vi "Log Data Core.vi"(8 "Error In":errorcluster, 10 "Log Message":T1={"Log Action"=enum."Handle Old Files", "Variant"=variant, "Data Type"=enum."String", "Group Name"="", "Channels Names"=[]}, 11 "TDMS Log In":refnum<class "TDMS Logger.lvclass">) -> (0 "Error Out":errorcluster, 3 "TDMS Log Out":refnum<class "TDMS Logger.lvclass">)   [LabVIEW 2015, in "TDMS Logger.lvlib" / "TDMS Logger.lvclass"]
uses:
  TDMS Logger.lvclass
  _Typedefs/Log Message.ctl
  _Typedefs/Log Action.ctl
  _Typedefs/Data Type.ctl
  TDMS Logger.lvclass/TDMS Logger.ctl
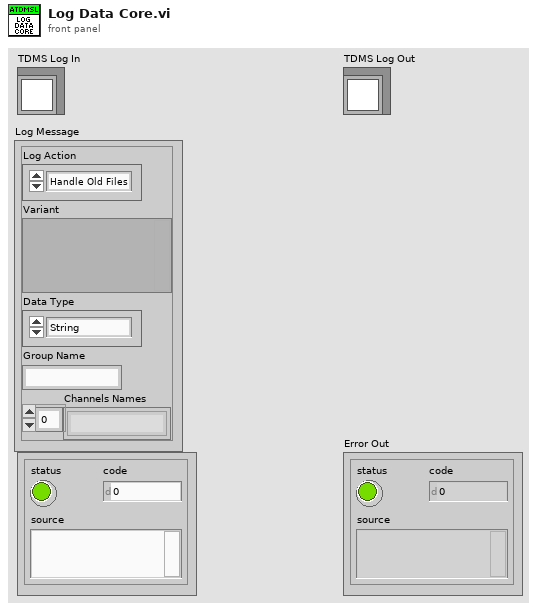
[diagram p1: front panel]
types:
  T1 = typedef "TDMS Logger.lvlib/TDMS Logger.lvclass/Log Message.ctl" = cluster{"Log Action":T2, "Variant":variant, "Data Type":T3, "Group Name":string, "Channels Names":string[]}
  T2 = typedef "TDMS Logger.lvlib/TDMS Logger.lvclass/Log Action.ctl" = enum16{"Handle Old Files", "Status Update", "Stop", "Log Data", "Initialize"}
  T3 = typedef "TDMS Logger.lvlib/TDMS Logger.lvclass/Data Type.ctl" = enum16{"I16", "I8", "String", "U16", "U8", "Waveform", "Double", "Single"}
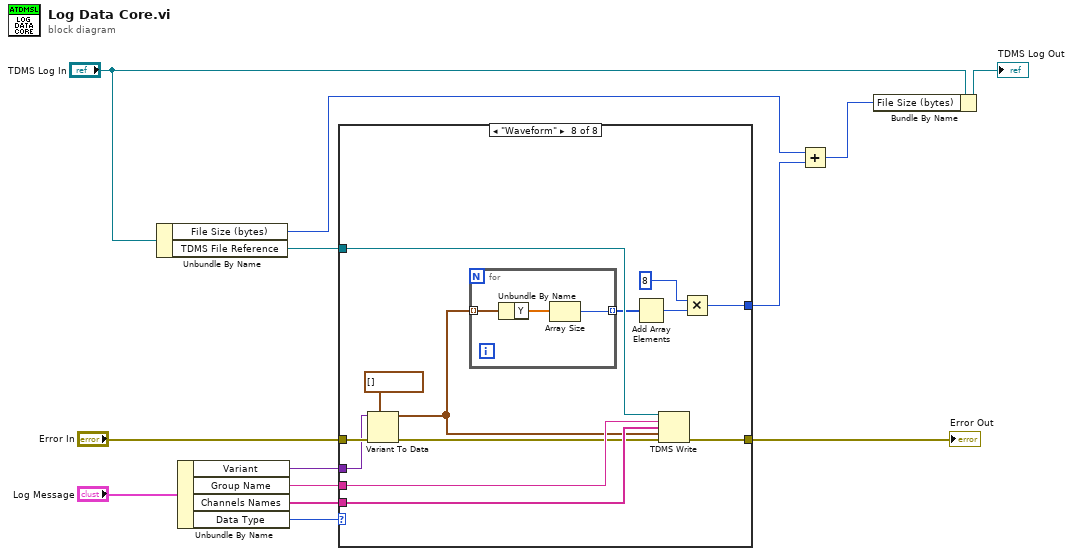
[diagram p0: block diagram]
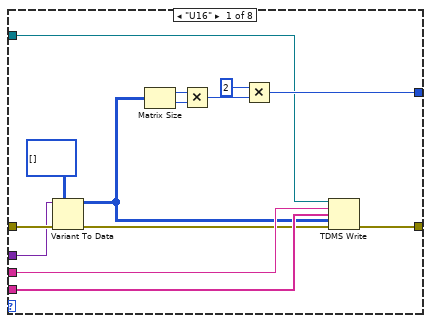
[diagram p2: hidden frame]
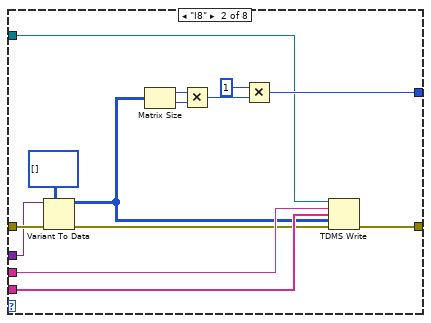
[diagram p3: hidden frame]
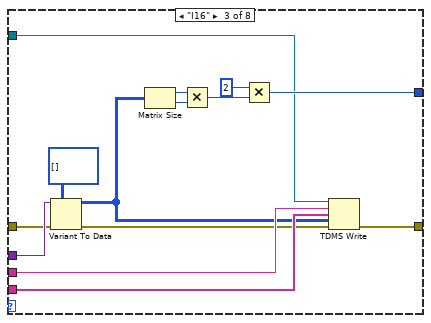
[diagram p4: hidden frame]
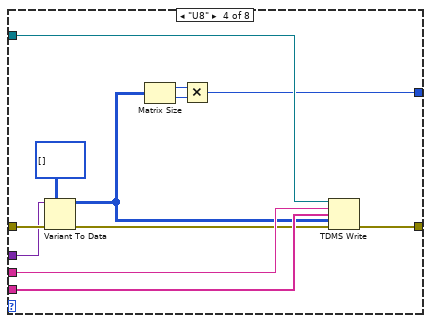
[diagram p5: hidden frame]
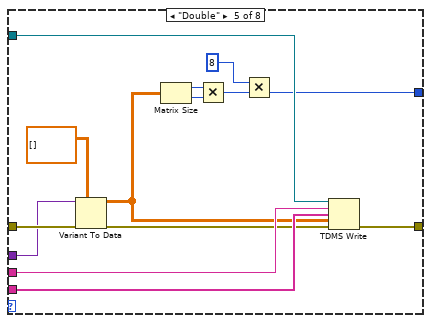
[diagram p6: hidden frame]
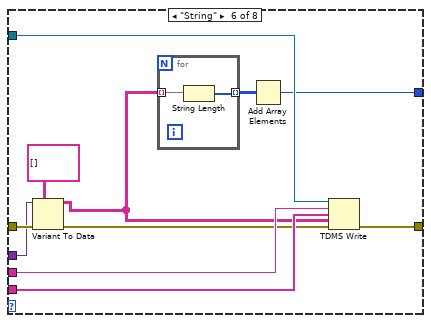
[diagram p7: hidden frame]
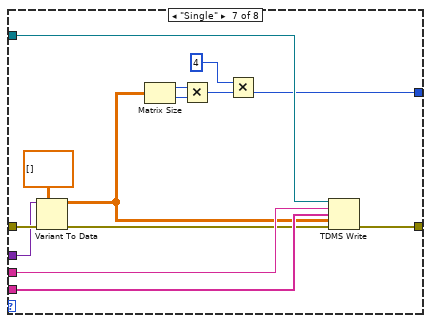
[diagram p8: hidden frame]
diagram:
  n1 = Unbundle By Name("TDMS Log In") -> ("File Size (bytes)"=w2:u64, "TDMS File Reference"=w4:refnum<k34>)
  n2 = Unbundle By Name("Log Message") -> ("Variant"=w1:variant, "Group Name"=w6:string, "Channels Names"=w5:string[], "Data Type"=w9:T3)
  n3 = case shown="\"Waveform\"" w9 {
    tunnel: "Error In" -> [w18 w32 w43 w60 w72 w86 w99 w113]
    tunnel: [w23 w41 w55 w61 w74 w87 w101 w117] -> w7
    tunnel: w6 -> [w22 w40 w54 w65 w79 w92 w106 w121]
    tunnel: w5 -> [w21 w39 w53 w64 w78 w91 w105 w120]
    tunnel: w4 -> [w20 w38 w52 w63 w77 w90 w104 w119]
    tunnel: [w19 w37 w51 w62 w76 w89 w103 w118] -> w3
    tunnel: w1 -> [w16 w28 w44 w56 w71 w82 w98 w109]
    frame "U16" {
      n4 = Variant To Data(error in=w18, type=u16[][] [] ("element"), Variant=w16) -> (data=w14:u16[][], error out=w17:errorcluster)
      n5 = Matrix Size(0:w14) -> (1:w25:i32, 2:w26:i32)
      n6 = Multiply(x=w25, y=w26) -> (x*y=w24:i32)
      n7 = Multiply(x=2, y=w24) -> (x*y=w23:i32)
      n8 = TDMS Write(0:w20, 5:w22, 7:w21, 9:w14, 11:w17) -> (15:w19:errorcluster)  [unwired: 1 in, 3 out]
    }
    frame "I8" {
      n9 = Variant To Data(error in=w32, type=i8[][] [] ("element"), Variant=w28) -> (data=w29:i8[][], error out=w31:errorcluster)
      n10 = Matrix Size(0:w29) -> (1:w34:i32, 2:w35:i32)
      n11 = Multiply(x=w34, y=w35) -> (x*y=w33:i32)
      n12 = Multiply(x=1, y=w33) -> (x*y=w41:i32)
      n13 = TDMS Write(0:w38, 5:w40, 7:w39, 9:w29, 11:w31) -> (15:w37:errorcluster)  [unwired: 1 in, 3 out]
    }
    frame "I16" {
      n14 = Variant To Data(error in=w43, type=i16[][] [] ("element"), Variant=w44) -> (data=w46:i16[][], error out=w42:errorcluster)
      n15 = Matrix Size(0:w46) -> (1:w48:i32, 2:w49:i32)
      n16 = Multiply(x=w48, y=w49) -> (x*y=w47:i32)
      n17 = Multiply(x=2, y=w47) -> (x*y=w55:i32)
      n18 = TDMS Write(0:w52, 5:w54, 7:w53, 9:w46, 11:w42) -> (15:w51:errorcluster)  [unwired: 1 in, 3 out]
    }
    frame "U8" {
      n19 = Variant To Data(error in=w60, type=u8[][] [] ("element"), Variant=w56) -> (data=w57:u8[][], error out=w59:errorcluster)
      n20 = Matrix Size(0:w57) -> (1:w66:i32, 2:w67:i32)
      n21 = Multiply(x=w66, y=w67) -> (x*y=w61:i32)
      n22 = TDMS Write(0:w63, 5:w65, 7:w64, 9:w57, 11:w59) -> (15:w62:errorcluster)  [unwired: 1 in, 3 out]
    }
    frame "Double" {
      n23 = Variant To Data(error in=w72, type=dbl[][] [], Variant=w71) -> (data=w68:dbl[][], error out=w70:errorcluster)
      n24 = Matrix Size(0:w68) -> (1:w80:i32, 2:w81:i32)
      n25 = Multiply(x=w80, y=w81) -> (x*y=w75:i32)
      n26 = Multiply(x=8, y=w75) -> (x*y=w74:i32)
      n27 = TDMS Write(0:w77, 5:w79, 7:w78, 9:w68, 11:w70) -> (15:w76:errorcluster)  [unwired: 1 in, 3 out]
    }
    frame "String" {
      n28 = Variant To Data(error in=w86, type=string[][] [] ("element"), Variant=w82) -> (data=w83:string[][], error out=w85:errorcluster)
      n29 = for {
        tunnel: w83 -> [w94] mode=indexing
        tunnel: [w93] -> w88 mode=indexing
        n30 = String Length(string=w94) -> (length=w93:i32[])
      }
      n31 = Add Array Elements(numeric array=w88) -> (sum=w87:i32)
      n32 = TDMS Write(0:w90, 5:w92, 7:w91, 9:w83, 11:w85) -> (15:w89:errorcluster)  [unwired: 1 in, 3 out]
    }
    frame "Single" {
      n33 = Variant To Data(error in=w99, type=sgl[][] [] ("element"), Variant=w98) -> (data=w95:sgl[][], error out=w96:errorcluster)
      n34 = Matrix Size(0:w95) -> (1:w107:i32, 2:w108:i32)
      n35 = Multiply(x=w107, y=w108) -> (x*y=w102:i32)
      n36 = Multiply(x=4, y=w102) -> (x*y=w101:i32)
      n37 = TDMS Write(0:w104, 5:w106, 7:w105, 9:w95, 11:w96) -> (15:w103:errorcluster)  [unwired: 1 in, 3 out]
    }
    frame "Waveform" {
      n38 = Variant To Data(error in=w113, type=waveform(dbl)[] [] ("element"), Variant=w109) -> (data=w110:waveform(dbl)[], error out=w112:errorcluster)
      n39 = for {
        tunnel: w110 -> [w124] mode=indexing
        tunnel: [w122] -> w114 mode=indexing
        n40 = Unbundle By Name(w124) -> ("Y"=w123:dbl[])
        n41 = Array Size(array=w123) -> (size(s)=w122:i32)
      }
      n42 = Add Array Elements(numeric array=w114) -> (sum=w115:i32)
      n43 = TDMS Write(0:w119, 5:w121, 7:w120, 9:w110, 11:w112) -> (15:w118:errorcluster)  [unwired: 1 in, 3 out]
      n44 = Multiply(x=8, y=w115) -> (x*y=w117:i32)
    }
  }
  "Error Out" <- w3
  n45 = Add(x=w2, y=w7) -> (x+y=w10:u64)
  n46 = Bundle By Name(cluster="TDMS Log In", "File Size (bytes)"=w10) -> (→"TDMS Log Out":refnum<class "TDMS Logger.lvclass">)
